vi "STM Read Message (UDP).vi"(6 "Options":T1={"Ignore Timeout Error"=TRUE, "timeout ms (1000)"=1000, "max size (548)"=548}, 8 "error in":errorcluster, 11 "Connection Info":T3) -> (0 "error out":errorcluster, 1 "Name":T4, 2 "data string":string, 3 "Connection Info Out":T3, 4 "Data Info":T2, 5 "Timed Out?":bool)   [LabVIEW 2014, in "QwaveSys Raspberry Pi Library.lvlib"]
doc: "This VI reads an incoming package of data from a host. This VI parses the package and extracts the data name and type as described in the meta data.\n\nFor the package to be parsed correctly, the meta data must be consistent in both the sender and the receiver. The data is packaged based on the existing meta data on the sender. \n\nUse the \"STM Read Meta Data\" and \"STM Write Meta Data\" VIs to ensure that both client and server have the same meta data.\n\nThe data is returned as a string. It is the responsibility of the user to cast it to the appropriate type."
uses:
  QwaveSys Raspberry Pi Library.lvlib
  _SubVIs/stm_MetaDataElement.ctl
  stm_UDP Connection Info.ctl
  stm_UDP Data Info.ctl
  stm_UDP Read Options.ctl
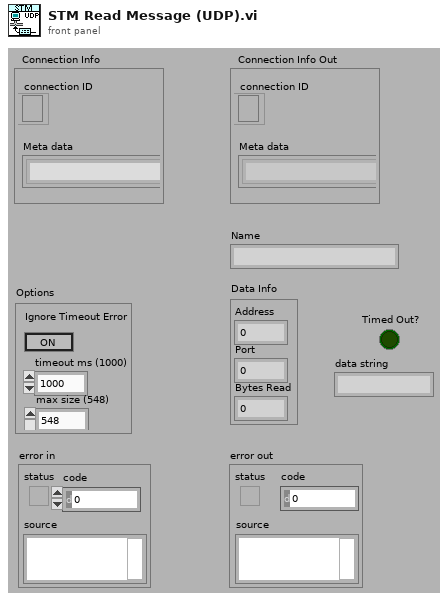
[diagram p1: front panel]
types:
  T1 = typedef "QwaveSys Raspberry Pi Library.lvlib/stm_UDP Read Options.ctl" = cluster{"Ignore Timeout Error":bool, "timeout ms (1000)":i32, "max size (548)":i32}
  T2 = typedef "QwaveSys Raspberry Pi Library.lvlib/stm_UDP Data Info.ctl" = cluster{"Address":u32, "Port":u16, "Bytes Read":i32}
  T3 = typedef "QwaveSys Raspberry Pi Library.lvlib/stm_UDP Connection Info.ctl" = cluster{"connection ID":refnum<k16>, "Meta data":T4[]}
  T4 = typedef "QwaveSys Raspberry Pi Library.lvlib/stm_MetaDataElement.ctl" = string
  T5 = cluster{"address":u32, "port":u16, "bytes to read":i32}
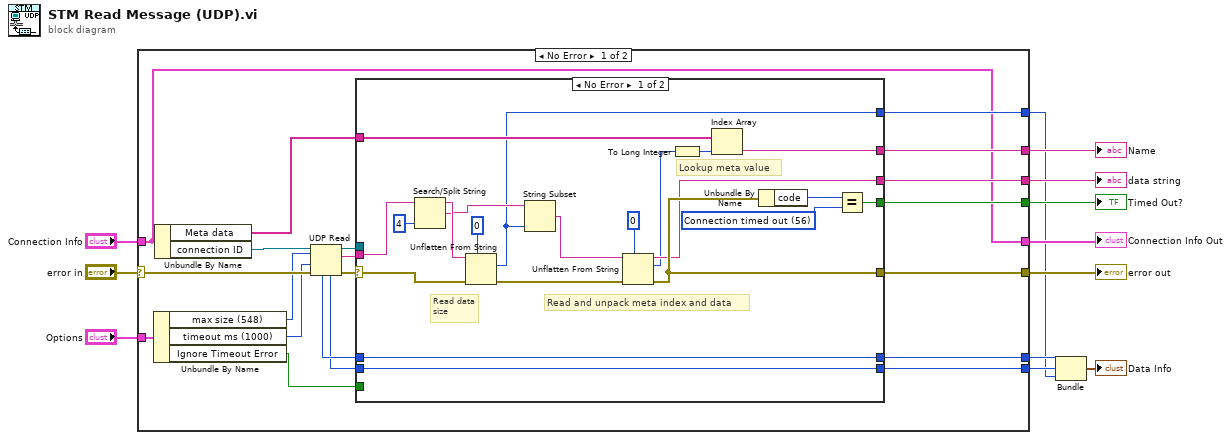
[diagram p0: block diagram]
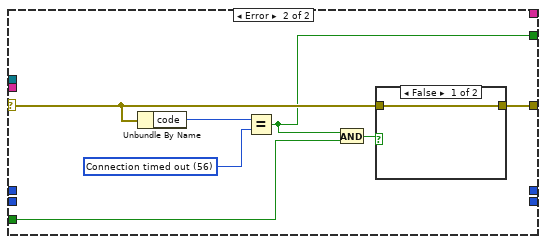
[diagram p2: hidden frame]
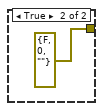
[diagram p3: hidden frame]
diagram:
  n1 = case shown="No Error" "error in" {
    selector: "error in" -> [w20 w63]
    tunnel: "Connection Info" -> [w13 w64]
    tunnel: [w13 w64] -> w7
    tunnel: [w32 w63] -> w12
    tunnel: [w31 _] -> w11
    tunnel: [w30 _] -> w10
    tunnel: [w29 _] -> w9
    tunnel: [w28 _] -> w4
    tunnel: [w23 _] -> w6
    tunnel: [w21 _] -> w5
    tunnel: "Options" -> [w19 _]
    frame No Error {
      n2 = Unbundle By Name(w19) -> ("max size (548)"=w17:i32, "timeout ms (1000)"=w16:i32, "Ignore Timeout Error"=w18:bool)
      n3 = Unbundle By Name(w13) -> ("Meta data"=w14:T4[], "connection ID"=w15:refnum<k16>)
      n4 = UDP Read(connection ID=w15, max size (548)=w17, timeout ms (25000)=w16, 8:w20) -> (data out=w25:string, error out=w27:errorcluster, 3:w26:refnum<k16>, 4:w22:u16, 6:w24:u32)
      n5 = case shown="No Error" w27 {
        selector: w27 -> [w49 w55]
        tunnel: w25 -> [w43 _]
        tunnel: w26 -> [_ _]
        tunnel: w14 -> [w53 _]
        tunnel: [w48 w56] -> w32
        tunnel: w18 -> [_ w58]
        tunnel: [w50 w54] -> w31
        tunnel: [w47 _] -> w30
        tunnel: [w35 _] -> w29
        tunnel: [w40 _] -> w28
        tunnel: [w38 _] -> w23
        tunnel: w24 -> [w38 _]
        tunnel: [w37 _] -> w21
        tunnel: w22 -> [w37 _]
        frame No Error {
          w51 = 56 items=["No Error", "Argument Error", "Memory Full", "Out of Zone", "End of File", "File Already Open", "Generic File IO Error", "File Not Found", "File Permission Error", "Disk Full", "Duplicate Path", "Too Many Files Open", "Not Enabled", "Resource File Not Found", "Cannot Add Resource", "Resource Not Found", "Image Not Found", "Image Memory Error", "Pen Does Not Exist", "Config Bad Type", "Config Token Not Found", "Config Parse Error", "Config Memory Error", "Bad External Code Format", "Bad External Code Offset", "External Code Not Present", "Null Window", "Destroy Window Mixup", "Null Menu", "Print Aborted", "Bad Print Record", "Print Driver Error", "Windows Error During Print", "Memory Error During Print", "Print Dialog Error", "Generic Print Error", "Invalid Device Refnum", "Device Not Found", "Device Parameter Error", "Device Unit Error", "Can't Open Device", "Device Call Aborted", "Generic Error", "Cancelled By User", "Object ID Too Low", "Object ID Too High", "Object Not In Heap", "Unknown Heap", "Bad DefProc ID", "DefProc Not In Table", "Message Out Of Range", "Null Method", "Unknown Message", "Manager Call Not Supported", "Bad address", "Connection In progress", "Connection timed out", "Connection is already in progress", "Network attribute not supported", "Network error", "Address in use", "System out of memory", "Connection aborted", "Connection refused", "Connection is not connected", "Connection is already connected", "Connection closed", "Initialize error (interapplication manager)", "Bad occurrence", "Wait on unbound occurrence handler", "Occurrence queue overflow", "Bad path", "Semaphore not signaled", "Unrecognized type (interapplication manager)"] ("1st Error to Convert")
          # "Read data size"
          # "Lookup meta value"
          # "Read and unpack meta index and data"
          n6 = Search/Split String(string=w43, offset (0)=4) -> (substring before match=w42:string, match + rest of string=w41:string)  [unwired: 2 out]
          n7 = Unflatten From String(type=0 ("bytes to read"), binary string=w42, error in (no error)=w49) -> (value=w40:i32, error out=w45:errorcluster)  [unwired: 1 in, 2 out]
          n8 = String Subset(string=w41, length (rest)=w40) -> (substring=w39:string)  [unwired: 1 out]
          n9 = Unflatten From String(type=u16 0, binary string=w39, error in (no error)=w45) -> (rest of the binary string=w35:string, value=w33:u16, error out=w48:errorcluster)  [unwired: 2 out]
          n10 = To Long Integer(number=w33) -> (32bit integer=w34:i32)
          n11 = Index Array(array=w53, index=w34) -> (element=w47:T4)
          n12 = Unbundle By Name(w48) -> ("code"=w52:i32)
          n13 = Equal?(x=w52, y=w51) -> (x = y?=w50:bool)
        }
        frame Error {
          w59 = 56 items=["No Error", "Argument Error", "Memory Full", "Out of Zone", "End of File", "File Already Open", "Generic File IO Error", "File Not Found", "File Permission Error", "Disk Full", "Duplicate Path", "Too Many Files Open", "Not Enabled", "Resource File Not Found", "Cannot Add Resource", "Resource Not Found", "Image Not Found", "Image Memory Error", "Pen Does Not Exist", "Config Bad Type", "Config Token Not Found", "Config Parse Error", "Config Memory Error", "Bad External Code Format", "Bad External Code Offset", "External Code Not Present", "Null Window", "Destroy Window Mixup", "Null Menu", "Print Aborted", "Bad Print Record", "Print Driver Error", "Windows Error During Print", "Memory Error During Print", "Print Dialog Error", "Generic Print Error", "Invalid Device Refnum", "Device Not Found", "Device Parameter Error", "Device Unit Error", "Can't Open Device", "Device Call Aborted", "Generic Error", "Cancelled By User", "Object ID Too Low", "Object ID Too High", "Object Not In Heap", "Unknown Heap", "Bad DefProc ID", "DefProc Not In Table", "Message Out Of Range", "Null Method", "Unknown Message", "Manager Call Not Supported", "Bad address", "Connection In progress", "Connection timed out", "Connection is already in progress", "Network attribute not supported", "Network error", "Address in use", "System out of memory", "Connection aborted", "Connection refused", "Connection is not connected", "Connection is already connected", "Connection closed", "Initialize error (interapplication manager)", "Bad occurrence", "Wait on unbound occurrence handler", "Occurrence queue overflow", "Bad path", "Semaphore not signaled", "Unrecognized type (interapplication manager)"] ("1st Error to Convert")
          n14 = Unbundle By Name(w55) -> ("code"=w60:i32)
          n15 = Equal?(x=w60, y=w59) -> (x = y?=w54:bool)
          n16 = And(x=w54, y=w58) -> (x .and. y?=w57:bool)
          n17 = case shown="False" w57 {
            tunnel: [w61 errorcluster {"status"=FALSE, "code"=0, "source"=""} ("error out")] -> w56
            tunnel: w55 -> [w61 _]
            frame False {
            }
            frame True {
            }
          }
        }
      }
    }
    frame Error {
    }
  }
  "error out" <- w12
  "Timed Out?" <- w11
  "data string" <- w9
  "Name" <- w10
  "Connection Info Out" <- w7
  n18 = Bundle("address"=w6, "port"=w5, "bytes to read"=w4) -> (→"Data Info":T5)  [unwired: 1 out]
